vi "exp_status.vi"() -> ()   [LabVIEW 2019, in "Global.lvlib"]
uses:
  Global.lvlib
panel:
  in  "Status":string="0"
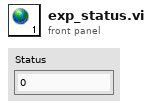
[diagram p1: front panel]
diagram:
